vi "Write DC Pins.vi"(8 "error in (no error)":errorcluster, 10 "DC Pins":string[](array[string]), 11 "DCLeakage in":refnum<class "DCLeakage.lvclass">) -> (0 "error out":errorcluster, 3 "DCLeakage out":refnum<class "DCLeakage.lvclass">)   [LabVIEW 2018, in "SeqAuto Evaluations.lvlib" / "DCLeakage.lvclass"]
uses:
  DCLeakage.lvclass
  DCLeakage.lvclass/DCLeakage.ctl
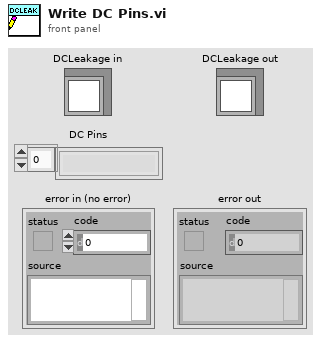
[diagram p1: front panel]
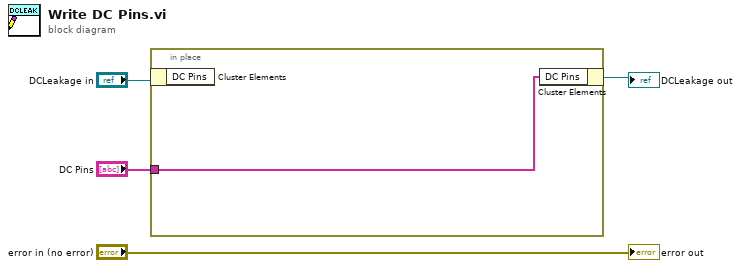
[diagram p0: block diagram]
diagram:
  n1 = in-place {
    in-place-border: "DC Pins" -> [w5]
    n2 = in-place-cluster #1("DCLeakage in") -> ()  [unwired: 1 out]
    n3 = in-place-cluster #1("DC Pins"=w5) -> (→"DCLeakage out":refnum<class "DCLeakage.lvclass">)
  }
  "error out" <- "error in (no error)"
